vi "split_trigger.vi"(6 "disable splitting":bool, 8 "N in":u32, 10 "trigger in":bool, 11 "counter in":u32) -> (0 "N out":u32, 2 "split trigger out":bool, 3 "counter out":u32)   [LabVIEW 2010]
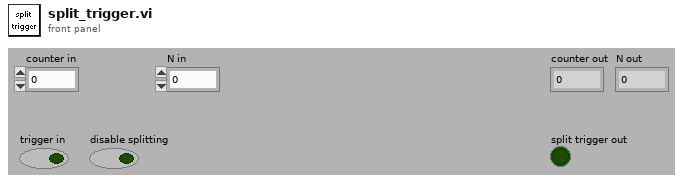
[diagram p1: front panel]
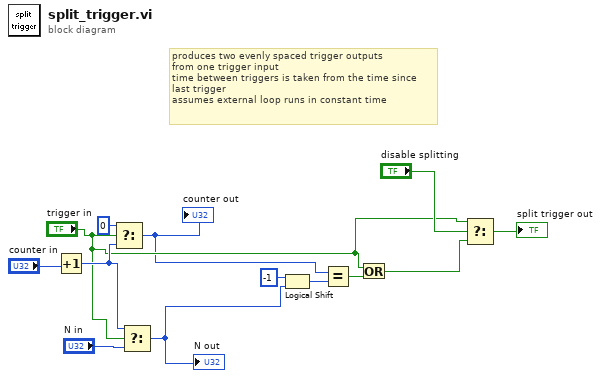
[diagram p0: block diagram]
diagram:
  # "produces two evenly spaced trigger outputs\nfrom one trigger input\ntime between triggers is taken from the time since\nlast trigger\nassumes external loop runs in constant time"
  n1 = Increment(x="counter in") -> (x+1=w7:u32)
  n2 = Select(t=u32 0, s="trigger in", f=w7) -> (s? t:f=w1:u32)
  "counter out" <- w1
  n3 = Select(t=w7, s="trigger in", f="N in") -> (s? t:f=w6:u32)
  "N out" <- w6
  n4 = Logical Shift(y=i16 -1 ("n"), x=w6) -> (x << y=w5:u32)
  n5 = Equal?(x=w1, y=w5) -> (x = y?=w4:bool)
  n6 = Or(x="trigger in", y=w4) -> (x .or. y?=w3:bool)
  n7 = Select(t="trigger in", s="disable splitting", f=w3) -> (s? t:f=→"split trigger out":bool)
